vi "User menu handler.vi"(9 "UI queue":refnum<queue>, 11 "User Menu ItemTag":string) -> (0 "error out":errorcluster)   [LabVIEW 2017]
uses:
  Queue/Message Queue/Typedefs/Message Cluster.ctl
  Global Variables/General Globals.vi
  Configuration code/Calibration/Globals/gl_Calibration globals.vi
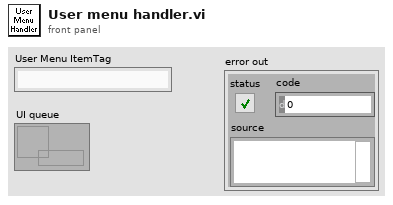
[diagram p1: front panel]
types:
  T1 = enum16{"Software Init", "User menu", "Switch User button"}
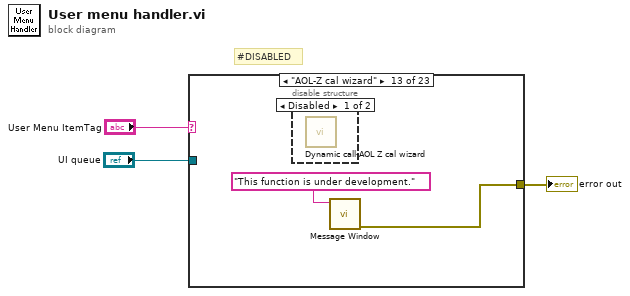
[diagram p0: block diagram]
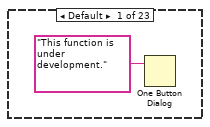
[diagram p2: hidden frame]
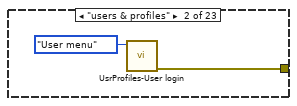
[diagram p3: hidden frame]
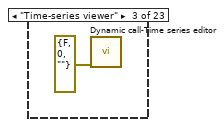
[diagram p4: hidden frame]
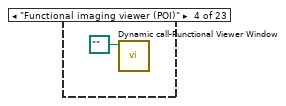
[diagram p5: hidden frame]
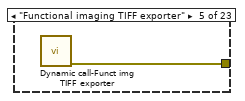
[diagram p6: hidden frame]
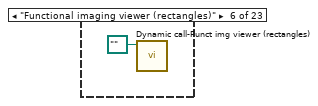
[diagram p7: hidden frame]
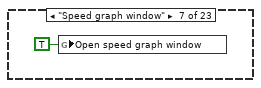
[diagram p8: hidden frame]
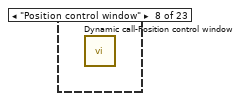
[diagram p9: hidden frame]
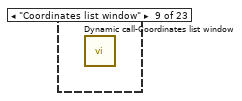
[diagram p10: hidden frame]
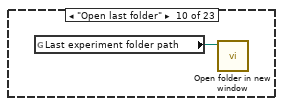
[diagram p11: hidden frame]
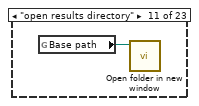
[diagram p12: hidden frame]
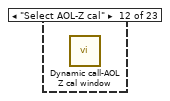
[diagram p13: hidden frame]
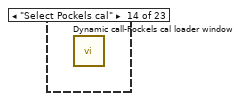
[diagram p15: hidden frame]
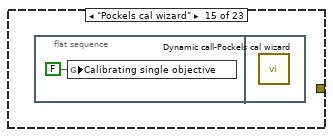
[diagram p16: hidden frame]
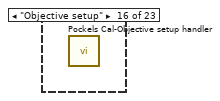
[diagram p17: hidden frame]
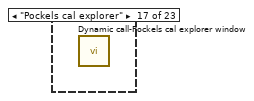
[diagram p18: hidden frame]
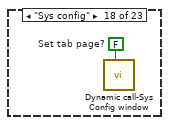
[diagram p19: hidden frame]
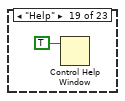
[diagram p20: hidden frame]
diagram:
  # "#DISABLED"
  n1 = case shown="\"AOL-Z cal wizard\"" "User Menu ItemTag" {
    tunnel: "UI queue" -> [_ _ _ _ _ _ _ _ _ _ _ _ _ _ _ _ _ _ _ _ _ w20 w22]
    tunnel: [_ w6 _ _ w9 _ _ _ _ _ _ _ w14 _ _ _ _ _ _ _ _ w19 w21] -> w1
    frame Default {
      n2 = One Button Dialog(message="This function is under development.") -> ()  [unwired: 1 in, 1 out]
    }
    frame "users & profiles" {
      n3 = call "UsrProfiles-User login.vi"("Access source (Soft init)"=T1."User menu") -> ("error out"=w6:errorcluster)  [unwired: 10 in]
    }
    frame "Time-series viewer" {
      n4 = call "Dynamic call-Time series editor.vi"("error in (no error)"=errorcluster {"status"=FALSE, "code"=0, "source"=""}) -> ()  [unwired: 10 in, 1 out]
    }
    frame "Functional imaging viewer (POI)" {
      n5 = call "Dynamic call-Functional Viewer Window.vi"("Experiment data folder path"=path "") -> ()  [unwired: 11 in]
    }
    frame "Functional imaging TIFF exporter" {
      n6 = call "Dynamic call-Funct img TIFF exporter.vi"() -> ("error out"=w9:errorcluster)  [unwired: 11 in]
    }
    frame "Functional imaging viewer (rectangles)" {
      n7 = call "Dynamic call-Funct img viewer (rectangles).vi"("Experiment Path"=path "") -> ()  [unwired: 10 in, 1 out]
    }
    frame "Speed graph window" {
      n8 = global write "General Globals.vi" "Open speed graph window"(TRUE ("Open speed graph window")) -> ()
    }
    frame "Position control window" {
      n9 = call "Dynamic call-Position control window.vi"() -> ()  [unwired: 11 in, 1 out]
    }
    frame "Coordinates list window" {
      n10 = call "Dynamic call-Coordinates list window.vi"() -> ()  [unwired: 11 in, 1 out]
    }
    frame "Open last folder" {
      n11 = global read "General Globals.vi" "Last experiment folder path"() -> (w12:path)
      n12 = call "Open folder in new window.vi"("Directory to open"=w12) -> ()  [unwired: 10 in, 1 out]
    }
    frame "open results directory" {
      n13 = global read "General Globals.vi" "Base path"() -> (w13:path)
      n14 = call "Open folder in new window.vi"("Directory to open"=w13) -> ()  [unwired: 10 in, 1 out]
    }
    frame "Select AOL-Z cal" {
      n15 = call "Dynamic call-AOL Z cal window.vi"() -> ()  [unwired: 11 in, 1 out]
    }
    frame "AOL-Z cal wizard" {
      n16 = disable-structure shown="Disabled" {
        frame Disabled {
          n17 = call "Dynamic call-AOL Z cal wizard.vi"() -> ()  [unwired: 11 in, 1 out]
        }
        frame Enabled {
        }
      }
      n18 = call "Message Window.vi"("Message string"="This function is under development.") -> ("error out (no error)"=w14:errorcluster)  [unwired: 10 in]
    }
    frame "Select Pockels cal" {
      n19 = call "Dynamic call-Pockels cal loader window.vi"() -> ()  [unwired: 11 in, 1 out]
    }
    frame "Pockels cal wizard" {
      n20 = flat-sequence {
        frame #0 {
          n21 = global write "gl_Calibration globals.vi" "Calibrating single objective"(FALSE ("Calibrating single objective")) -> ()
        }
        frame #1 {
          n22 = call "Dynamic call-Pockels cal wizard.vi"() -> ()  [unwired: 11 in, 1 out]
        }
      }
    }
    frame "Objective setup" {
      n23 = call "Pockels Cal-Objective setup handler.vi"() -> ()  [unwired: 12 in]
    }
    frame "Pockels cal explorer" {
      n24 = call "Dynamic call-Pockels cal explorer window.vi"() -> ()  [unwired: 11 in, 1 out]
    }
    frame "Sys config" {
      w17 = FALSE  # Set tab page?
      n25 = call "Dynamic call-Sys Config window.vi"("Set tab page? (F)"=w17) -> ()  [unwired: 10 in, 1 out]
    }
    frame "Help" {
      n26 = Control Help Window(1:TRUE ("Show")) -> ()  [unwired: 1 in]
    }
    frame "Web" {
      n27 = call "SilverLab Web.vi"() -> ()  [unwired: 12 in]
    }
    frame "About" {
      n28 = call "Window-About.vi"() -> ()  [unwired: 12 in]
    }
    frame "shut down" {
      n29 = disable-structure shown="Disabled" {
        frame Disabled {
          n30 = call "Window-Exit window.vi"() -> ()  [unwired: 10 in, 2 out]
        }
        frame Enabled {
        }
      }
      n31 = call "Event handler-Exit.vi"("UI queue"=w20) -> ("error out"=w19:errorcluster)  [unwired: 9 in, 1 out]
    }
    frame "restart" {
      n32 = disable-structure shown="Disabled" {
        frame Disabled {
          n33 = call "Window-Restart window.vi"() -> ()  [unwired: 10 in, 2 out]
        }
        frame Enabled {
        }
      }
      n34 = call "Event handler-Restart.vi"("Queue in"=w22) -> ("error out"=w21:errorcluster)  [unwired: 10 in]
    }
  }
  "error out" <- w1
